vi "XIPIN_AXI_Virtual_FIFO_Controller_1_1.vi"   [LabVIEW 2017]
doc: "Rev 1. The AXI Virtual FIFO Controller is a parameterizable number of multi channel FIFO.\n------------------------------------\n<b>Need License</b> : No\n<b>Interface</b> : AXI4 AXI4-Stream"
uses:
  <vilib>/rvi/XilinxIP/XIPIN_XNode/niFpgaXIPIN.xnode
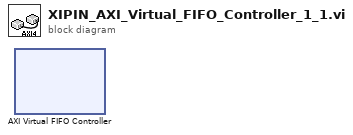
[diagram p0: block diagram]
diagram:
  n1 = xnode ("AXI Virtual FIFO Controller")() -> ()
